vi "Get SMO RC Type.vi"(8 "error in (no error)":errorcluster, 11 "Instrument in":refnum<class "Instrument.lvclass">) -> (0 "error out":errorcluster, 2 "RemoteControl":refnum<class "RemoteControl.lvclass">, 3 "Instrument out":refnum<class "Instrument.lvclass">)   [LabVIEW 2019, in "Instrument.lvlib" / "Instrument.lvclass"]
doc: "Override this VI to return the type of RemoteControl process used by your Instrument. The default is RemoteControl.ZMQ"
uses:
  Instrument.lvclass
  <userlib>/LevyLab/RemoteControl/RemoteControl/RemoteControl.lvclass
  <userlib>/LevyLab/RemoteControl.ZMQ/RemoteControl.ZMQ/RemoteControl.ZMQ.lvclass
  C:/Program Files (x86)/National Instruments/LabVIEW 2019/user.lib/LevyLab/RemoteControl/RemoteControl/RemoteControl.lvclass
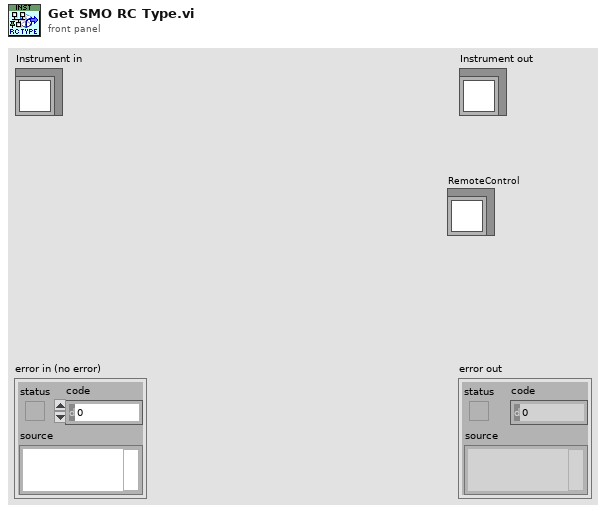
[diagram p1: front panel]
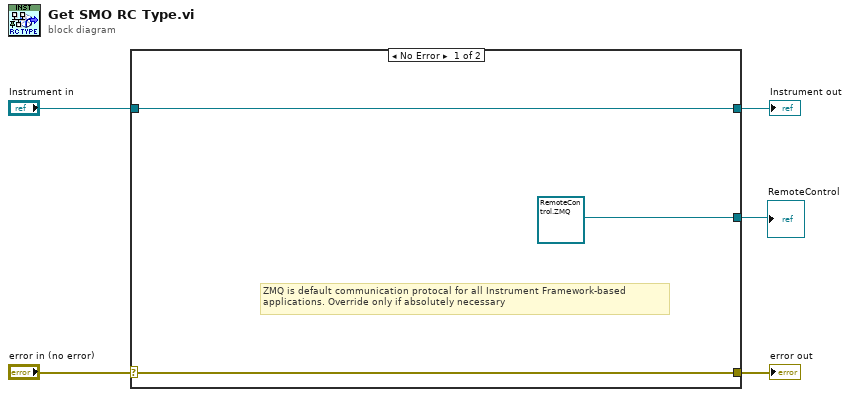
[diagram p0: block diagram]
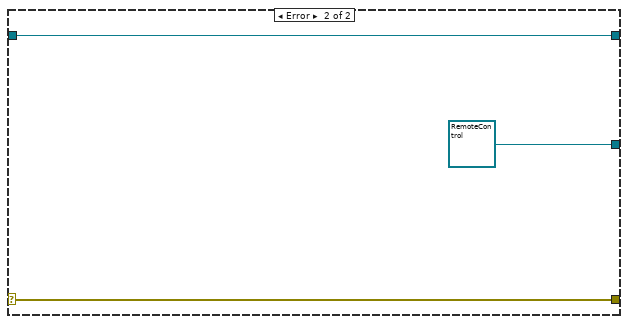
[diagram p2: hidden frame]
diagram:
  n1 = case shown="No Error" "error in (no error)" {
    selector: "error in (no error)" -> [w8 w11]
    tunnel: [w8 w11] -> w4
    tunnel: [w6 w10] -> w2
    tunnel: "Instrument in" -> [w6 w10]
    tunnel: [refnum<class "RemoteControl.ZMQ.lvclass"> refnum ("RemoteControl.ZMQ.lvlib:RemoteControl.ZMQ.lvclass") refnum<class "RemoteControl.lvclass"> refnum ("RemoteControl")] -> w1
    frame No Error {
      # "ZMQ is default communication protocal for all Instrument Framework-based\napplications. Override only if absolutely necessary"
    }
    frame Error {
    }
  }
  "error out" <- w4
  "Instrument out" <- w2
  "RemoteControl" <- w1
